vi "App - analyze RUS V6.vi"() -> ()   [LabVIEW 2021] (continued)
"last mod"=timestamp(3493836728 s since 1904-01-01), "file name str"="D:\\Data\\Ultrasound\\LSCO\\LSCO22__130814c\\5_Cooling_2nd_try\\September_2014\\091714\\27.11300K_500_2500_2.10000V_0.00000T_Sep17-2014__18-12-08_001_091714.bin", "mod time(min)"=58230612.13333333, "file format"=enum."binary", "power(V)"=2.1, "Magn Field(T) "=0.0}, {"temperature"=27.012, "temperature str"="27.01200", "file path"=path "D:/Data/Ultrasound/LSCO/LSCO22__130814c/5_Cooling_2nd_try/September_2014/091714/27.01200K_500_2500_2.10000V_0.00000T_Sep17-2014__18-13-27_001_091714.bin", "last mod"=timestamp(3493836807 s since 1904-01-01), "file name str"="D:\\Data\\Ultrasound\\LSCO\\LSCO22__130814c\\5_Cooling_2nd_try\\September_2014\\091714\\27.01200K_500_2500_2.10000V_0.00000T_Sep17-2014__18-13-27_001_091714.bin", "mod time(min)"=58230613.45, "file format"=enum."binary", "power(V)"=2.1, "Magn Field(T) "=0.0}, {"temperature"=26.919, "temperature str"="26.91900", "file path"=path "D:/Data/Ultrasound/LSCO/LSCO22__130814c/5_Cooling_2nd_try/September_2014/091714/26.91900K_500_2500_2.10000V_0.00000T_Sep17-2014__18-14-46_001_091714.bin", "last mod"=timestamp(3493836886 s since 1904-01-01), "file name str"="D:\\Data\\Ultrasound\\LSCO\\LSCO22__130814c\\5_Cooling_2nd_try\\September_2014\\091714\\26.91900K_500_2500_2.10000V_0.00000T_Sep17-2014__18-14-46_001_091714.bin", "mod time(min)"=58230614.766666666, "file format"=enum."binary", "power(V)"=2.1, "Magn Field(T) "=0.0}, {"temperature"=26.829, "temperature str"="26.82900", "file path"=path "D:/Data/Ultrasound/LSCO/LSCO22__130814c/5_Cooling_2nd_try/September_2014/091714/26.82900K_500_2500_2.10000V_0.00000T_Sep17-2014__18-16-06_001_091714.bin", "last mod"=timestamp(3493836966 s since 1904-01-01), "file name str"="D:\\Data\\Ultrasound\\LSCO\\LSCO22__130814c\\5_Cooling_2nd_try\\September_2014\\091714\\26.82900K_500_2500_2.10000V_0.00000T_Sep17-2014__18-16-06_001_091714.bin", "mod time(min)"=58230616.1, "file format"=enum."binary", "power(V)"=2.1, "Magn Field(T) "=0.0}, {"temperature"=26.729, "temperature str"="26.72900", "file path"=path "D:/Data/Ultrasound/LSCO/LSCO22__130814c/5_Cooling_2nd_try/September_2014/091714/26.72900K_500_2500_2.10000V_0.00000T_Sep17-2014__18-17-25_001_091714.bin", "last mod"=timestamp(3493837045 s since 1904-01-01), "file name str"="D:\\Data\\Ultrasound\\LSCO\\LSCO22__130814c\\5_Cooling_2nd_try\\September_2014\\091714\\26.72900K_500_2500_2.10000V_0.00000T_Sep17-2014__18-17-25_001_091714.bin", "mod time(min)"=58230617.416666664, "file format"=enum."binary", "power(V)"=2.1, "Magn Field(T) "=0.0}, {"temperature"=26.631, "temperature str"="26.63100", "file path"=path "D:/Data/Ultrasound/LSCO/LSCO22__130814c/5_Cooling_2nd_try/September_2014/091714/26.63100K_500_2500_2.10000V_0.00000T_Sep17-2014__18-18-44_001_091714.bin", "last mod"=timestamp(3493837124 s since 1904-01-01), "file name str"="D:\\Data\\Ultrasound\\LSCO\\LSCO22__130814c\\5_Cooling_2nd_try\\September_2014\\091714\\26.63100K_500_2500_2.10000V_0.00000T_Sep17-2014__18-18-44_001_091714.bin", "mod time(min)"=58230618.733333334, "file format"=enum."binary", "power(V)"=2.1, "Magn Field(T) "=0.0}, {"temperature"=26.532, "temperature str"="26.53200", "file path"=path "D:/Data/Ultrasound/LSCO/LSCO22__130814c/5_Cooling_2nd_try/September_2014/091714/26.53200K_500_2500_2.10000V_0.00000T_Sep17-2014__18-20-04_001_091714.bin", "last mod"=timestamp(3493837204 s since 1904-01-01), "file name str"="D:\\Data\\Ultrasound\\LSCO\\LSCO22__130814c\\5_Cooling_2nd_try\\September_2014\\091714\\26.53200K_500_2500_2.10000V_0.00000T_Sep17-2014__18-20-04_001_091714.bin", "mod time(min)"=58230620.06666667, "file format"=enum."binary", "power(V)"=2.1, "Magn Field(T) "=0.0}, {"temperature"=26.444, "temperature str"="26.44400", "file path"=path "D:/Data/Ultrasound/LSCO/LSCO22__130814c/5_Cooling_2nd_try/September_2014/091714/26.44400K_500_2500_2.10000V_0.00000T_Sep17-2014__18-21-23_001_091714.bin", "last mod"=timestamp(3493837283 s since 1904-01-01), "file name str"="D:\\Data\\Ultrasound\\LSCO\\LSCO22__130814c\\5_Cooling_2nd_try\\September_2014\\091714\\26.44400K_500_2500_2.10000V_0.00000T_Sep17-2014__18-21-23_001_091714.bin", "mod time(min)"=58230621.38333333, "file format"=enum."binary", "power(V)"=2.1, "Magn Field(T) "=0.0}, {"temperature"=26.344, "temperature str"="26.34400", "file path"=path "D:/Data/Ultrasound/LSCO/LSCO22__130814c/5_Cooling_2nd_try/September_2014/091714/26.34400K_500_2500_2.10000V_0.00000T_Sep17-2014__18-22-43_001_091714.bin", "last mod"=timestamp(3493837363 s since 1904-01-01), "file name str"="D:\\Data\\Ultrasound\\LSCO\\LSCO22__130814c\\5_Cooling_2nd_try\\September_2014\\091714\\26.34400K_500_2500_2.10000V_0.00000T_Sep17-2014__18-22-43_001_091714.bin", "mod time(min)"=58230622.71666667, "file format"=enum."binary", "power(V)"=2.1, "Magn Field(T) "=0.0}, {"temperature"=26.256, "temperature str"="26.25600", "file path"=path "D:/Data/Ultrasound/LSCO/LSCO22__130814c/5_Cooling_2nd_try/September_2014/091714/26.25600K_500_2500_2.10000V_0.00000T_Sep17-2014__18-24-02_001_091714.bin", "last mod"=timestamp(3493837442 s since 1904-01-01), "file name str"="D:\\Data\\Ultrasound\\LSCO\\LSCO22__130814c\\5_Cooling_2nd_try\\September_2014\\091714\\26.25600K_500_2500_2.10000V_0.00000T_Sep17-2014__18-24-02_001_091714.bin", "mod time(min)"=58230624.03333333, "file format"=enum."binary", "power(V)"=2.1, "Magn Field(T) "=0.0}, {"temperature"=26.156, "temperature str"="26.15600", "file path"=path "D:/Data/Ultrasound/LSCO/LSCO22__130814c/5_Cooling_2nd_try/September_2014/091714/26.15600K_500_2500_2.10000V_0.00000T_Sep17-2014__18-25-21_001_091714.bin", "last mod"=timestamp(3493837521 s since 1904-01-01), "file name str"="D:\\Data\\Ultrasound\\LSCO\\LSCO22__130814c\\5_Cooling_2nd_try\\September_2014\\091714\\26.15600K_500_2500_2.10000V_0.00000T_Sep17-2014__18-25-21_001_091714.bin", "mod time(min)"=58230625.35, "file format"=enum."binary", "power(V)"=2.1, "Magn Field(T) "=0.0}, {"temperature"=26.051, "temperature str"="26.05100", "file path"=path "D:/Data/Ultrasound/LSCO/LSCO22__130814c/5_Cooling_2nd_try/September_2014/091714/26.05100K_500_2500_2.10000V_0.00000T_Sep17-2014__18-26-41_001_091714.bin", "last mod"=timestamp(3493837601 s since 1904-01-01), "file name str"="D:\\Data\\Ultrasound\\LSCO\\LSCO22__130814c\\5_Cooling_2nd_try\\September_2014\\091714\\26.05100K_500_2500_2.10000V_0.00000T_Sep17-2014__18-26-41_001_091714.bin", "mod time(min)"=58230626.68333333, "file format"=enum."binary", "power(V)"=2.1, "Magn Field(T) "=0.0}, {"temperature"=25.961, "temperature str"="25.96100", "file path"=path "D:/Data/Ultrasound/LSCO/LSCO22__130814c/5_Cooling_2nd_try/September_2014/091714/25.96100K_500_2500_2.10000V_0.00000T_Sep17-2014__18-28-00_001_091714.bin", "last mod"=timestamp(3493837680 s since 1904-01-01), "file name str"="D:\\Data\\Ultrasound\\LSCO\\LSCO22__130814c\\5_Cooling_2nd_try\\September_2014\\091714\\25.96100K_500_2500_2.10000V_0.00000T_Sep17-2014__18-28-00_001_091714.bin", "mod time(min)"=58230628.0, "file format"=enum."binary", "power(V)"=2.1, "Magn Field(T) "=0.0}, {"temperature"=25.864, "temperature str"="25.86400", "file path"=path "D:/Data/Ultrasound/LSCO/LSCO22__130814c/5_Cooling_2nd_try/September_2014/091714/25.86400K_500_2500_2.10000V_0.00000T_Sep17-2014__18-29-20_001_091714.bin", "last mod"=timestamp(3493837760 s since 1904-01-01), "file name str"="D:\\Data\\Ultrasound\\LSCO\\LSCO22__130814c\\5_Cooling_2nd_try\\September_2014\\091714\\25.86400K_500_2500_2.10000V_0.00000T_Sep17-2014__18-29-20_001_091714.bin", "mod time(min)"=58230629.333333336, "file format"=enum."binary", "power(V)"=2.1, "Magn Field(T) "=0.0}, {"temperature"=25.765, "temperature str"="25.76500", "file path"=path "D:/Data/Ultrasound/LSCO/LSCO22__130814c/5_Cooling_2nd_try/September_2014/091714/25.76500K_500_2500_2.10000V_0.00000T_Sep17-2014__18-30-39_001_091714.bin", "last mod"=timestamp(3493837839 s since 1904-01-01), "file name str"="D:\\Data\\Ultrasound\\LSCO\\LSCO22__130814c\\5_Cooling_2nd_try\\September_2014\\091714\\25.76500K_500_2500_2.10000V_0.00000T_Sep17-2014__18-30-39_001_091714.bin", "mod time(min)"=58230630.65, "file format"=enum."binary", "power(V)"=2.1, "Magn Field(T) "=0.0}, {"temperature"=25.672, "temperature str"="25.67200", "file path"=path "D:/Data/Ultrasound/LSCO/LSCO22__130814c/5_Cooling_2nd_try/September_2014/091714/25.67200K_500_2500_2.10000V_0.00000T_Sep17-2014__18-31-58_001_091714.bin", "last mod"=timestamp(3493837918 s since 1904-01-01), "file name str"="D:\\Data\\Ultrasound\\LSCO\\LSCO22__130814c\\5_Cooling_2nd_try\\September_2014\\091714\\25.67200K_500_2500_2.10000V_0.00000T_Sep17-2014__18-31-58_001_091714.bin", "mod time(min)"=58230631.96666667, "file format"=enum."binary", "power(V)"=2.1, "Magn Field(T) "=0.0}, {"temperature"=25.576, "temperature str"="25.57600", "file path"=path "D:/Data/Ultrasound/LSCO/LSCO22__130814c/5_Cooling_2nd_try/September_2014/091714/25.57600K_500_2500_2.10000V_0.00000T_Sep17-2014__18-33-18_001_091714.bin", "last mod"=timestamp(3493837998 s since 1904-01-01), "file name str"="D:\\Data\\Ultrasound\\LSCO\\LSCO22__130814c\\5_Cooling_2nd_try\\September_2014\\091714\\25.57600K_500_2500_2.10000V_0.00000T_Sep17-2014__18-33-18_001_091714.bin", "mod time(min)"=58230633.3, "file format"=enum."binary", "power(V)"=2.1, "Magn Field(T) "=0.0}, {"temperature"=25.474, "temperature str"="25.47400", "file path"=path "D:/Data/Ultrasound/LSCO/LSCO22__130814c/5_Cooling_2nd_try/September_2014/091714/25.47400K_500_2500_2.10000V_0.00000T_Sep17-2014__18-34-37_001_091714.bin", "last mod"=timestamp(3493838077 s since 1904-01-01), "file name str"="D:\\Data\\Ultrasound\\LSCO\\LSCO22__130814c\\5_Cooling_2nd_try\\September_2014\\091714\\25.47400K_500_2500_2.10000V_0.00000T_Sep17-2014__18-34-37_001_091714.bin", "mod time(min)"=58230634.61666667, "file format"=enum."binary", "power(V)"=2.1, "Magn Field(T) "=0.0}, {"temperature"=25.388, "temperature str"="25.38800", "file path"=path "D:/Data/Ultrasound/LSCO/LSCO22__130814c/5_Cooling_2nd_try/September_2014/091714/25.38800K_500_2500_2.10000V_0.00000T_Sep17-2014__18-35-56_001_091714.bin", "last mod"=timestamp(3493838156 s since 1904-01-01), "file name str"="D:\\Data\\Ultrasound\\LSCO\\LSCO22__130814c\\5_Cooling_2nd_try\\September_2014\\091714\\25.38800K_500_2500_2.10000V_0.00000T_Sep17-2014__18-35-56_001_091714.bin", "mod time(min)"=58230635.93333333, "file format"=enum."binary", "power(V)"=2.1, "Magn Field(T) "=0.0}, {"temperature"=25.289, "temperature str"="25.28900", "file path"=path "D:/Data/Ultrasound/LSCO/LSCO22__130814c/5_Cooling_2nd_try/September_2014/091714/25.28900K_500_2500_2.10000V_0.00000T_Sep17-2014__18-37-16_001_091714.bin", "last mod"=timestamp(3493838236 s since 1904-01-01), "file name str"="D:\\Data\\Ultrasound\\LSCO\\LSCO22__130814c\\5_Cooling_2nd_try\\September_2014\\091714\\25.28900K_500_2500_2.10000V_0.00000T_Sep17-2014__18-37-16_001_091714.bin", "mod time(min)"=58230637.266666666, "file format"=enum."binary", "power(V)"=2.1, "Magn Field(T) "=0.0}, {"temperature"=25.188, "temperature str"="25.18800", "file path"=path "D:/Data/Ultrasound/LSCO/LSCO22__130814c/5_Cooling_2nd_try/September_2014/091714/25.18800K_500_2500_2.10000V_0.00000T_Sep17-2014__18-38-35_001_091714.bin", "last mod"=timestamp(3493838315 s since 1904-01-01), "file name str"="D:\\Data\\Ultrasound\\LSCO\\LSCO22__130814c\\5_Cooling_2nd_try\\September_2014\\091714\\25.18800K_500_2500_2.10000V_0.00000T_Sep17-2014__18-38-35_001_091714.bin", "mod time(min)"=58230638.583333336, "file format"=enum."binary", "power(V)"=2.1, "Magn Field(T) "=0.0}, {"temperature"=25.098, "temperature str"="25.09800", "file path"=path "D:/Data/Ultrasound/LSCO/LSCO22__130814c/5_Cooling_2nd_try/September_2014/091714/25.09800K_500_2500_2.10000V_0.00000T_Sep17-2014__18-39-55_001_091714.bin", "last mod"=timestamp(3493838395 s since 1904-01-01), "file name str"="D:\\Data\\Ultrasound\\LSCO\\LSCO22__130814c\\5_Cooling_2nd_try\\September_2014\\091714\\25.09800K_500_2500_2.10000V_0.00000T_Sep17-2014__18-39-55_001_091714.bin", "mod time(min)"=58230639.916666664, "file format"=enum."binary", "power(V)"=2.1, "Magn Field(T) "=0.0}, {"temperature"=24.995, "temperature str"="24.99500", "file path"=path "D:/Data/Ultrasound/LSCO/LSCO22__130814c/5_Cooling_2nd_try/September_2014/091714/24.99500K_500_2500_2.10000V_0.00000T_Sep17-2014__18-41-14_001_091714.bin", "last mod"=timestamp(3493838474 s since 1904-01-01), "file name str"="D:\\Data\\Ultrasound\\LSCO\\LSCO22__130814c\\5_Cooling_2nd_try\\September_2014\\091714\\24.99500K_500_2500_2.10000V_0.00000T_Sep17-2014__18-41-14_001_091714.bin", "mod time(min)"=58230641.233333334, "file format"=enum."binary", "power(V)"=2.1, "Magn Field(T) "=0.0}, {"temperature"=24.901, "temperature str"="24.90100", "file path"=path "D:/Data/Ultrasound/LSCO/LSCO22__130814c/5_Cooling_2nd_try/September_2014/091714/24.90100K_500_2500_2.10000V_0.00000T_Sep17-2014__18-42-33_001_091714.bin", "last mod"=timestamp(3493838553 s since 1904-01-01), "file name str"="D:\\Data\\Ultrasound\\LSCO\\LSCO22__130814c\\5_Cooling_2nd_try\\September_2014\\091714\\24.90100K_500_2500_2.10000V_0.00000T_Sep17-2014__18-42-33_001_091714.bin", "mod time(min)"=58230642.55, "file format"=enum."binary", "power(V)"=2.1, "Magn Field(T) "=0.0}, {"temperature"=24.798, "temperature str"="24.79800", "file path"=path "D:/Data/Ultrasound/LSCO/LSCO22__130814c/5_Cooling_2nd_try/September_2014/091714/24.79800K_500_2500_2.10000V_0.00000T_Sep17-2014__18-43-53_001_091714.bin", "last mod"=timestamp(3493838633 s since 1904-01-01), "file name str"="D:\\Data\\Ultrasound\\LSCO\\LSCO22__130814c\\5_Cooling_2nd_try\\September_2014\\091714\\24.79800K_500_2500_2.10000V_0.00000T_Sep17-2014__18-43-53_001_091714.bin", "mod time(min)"=58230643.88333333, "file format"=enum."binary", "power(V)"=2.1, "Magn Field(T) "=0.0}, {"temperature"=24.697, "temperature str"="24.69700", "file path"=path "D:/Data/Ultrasound/LSCO/LSCO22__130814c/5_Cooling_2nd_try/September_2014/091714/24.69700K_500_2500_2.10000V_0.00000T_Sep17-2014__18-45-12_001_091714.bin", "last mod"=timestamp(3493838712 s since 1904-01-01), "file name str"="D:\\Data\\Ultrasound\\LSCO\\LSCO22__130814c\\5_Cooling_2nd_try\\September_2014\\091714\\24.69700K_500_2500_2.10000V_0.00000T_Sep17-2014__18-45-12_001_091714.bin", "mod time(min)"=58230645.2, "file format"=enum."binary", "power(V)"=2.1, "Magn Field(T) "=0.0}, {"temperature"=24.601, "temperature str"="24.60100", "file path"=path "D:/Data/Ultrasound/LSCO/LSCO22__130814c/5_Cooling_2nd_try/September_2014/091714/24.60100K_500_2500_2.10000V_0.00000T_Sep17-2014__18-46-31_001_091714.bin", "last mod"=timestamp(3493838791 s since 1904-01-01), "file name str"="D:\\Data\\Ultrasound\\LSCO\\LSCO22__130814c\\5_Cooling_2nd_try\\September_2014\\091714\\24.60100K_500_2500_2.10000V_0.00000T_Sep17-2014__18-46-31_001_091714.bin", "mod time(min)"=58230646.516666666, "file format"=enum."binary", "power(V)"=2.1, "Magn Field(T) "=0.0}, {"temperature"=24.516, "temperature str"="24.51600", "file path"=path "D:/Data/Ultrasound/LSCO/LSCO22__130814c/5_Cooling_2nd_try/September_2014/091714/24.51600K_500_2500_2.10000V_0.00000T_Sep17-2014__18-47-51_001_091714.bin", "last mod"=timestamp(3493838871 s since 1904-01-01), "file name str"="D:\\Data\\Ultrasound\\LSCO\\LSCO22__130814c\\5_Cooling_2nd_try\\September_2014\\091714\\24.51600K_500_2500_2.10000V_0.00000T_Sep17-2014__18-47-51_001_091714.bin", "mod time(min)"=58230647.85, "file format"=enum."binary", "power(V)"=2.1, "Magn Field(T) "=0.0}, {"temperature"=24.408, "temperature str"="24.40800", "file path"=path "D:/Data/Ultrasound/LSCO/LSCO22__130814c/5_Cooling_2nd_try/September_2014/091714/24.40800K_500_2500_2.10000V_0.00000T_Sep17-2014__18-49-10_001_091714.bin", "last mod"=timestamp(3493838950 s since 1904-01-01), "file name str"="D:\\Data\\Ultrasound\\LSCO\\LSCO22__130814c\\5_Cooling_2nd_try\\September_2014\\091714\\24.40800K_500_2500_2.10000V_0.00000T_Sep17-2014__18-49-10_001_091714.bin", "mod time(min)"=58230649.166666664, "file format"=enum."binary", "power(V)"=2.1, "Magn Field(T) "=0.0}, {"temperature"=24.313, "temperature str"="24.31300", "file path"=path "D:/Data/Ultrasound/LSCO/LSCO22__130814c/5_Cooling_2nd_try/September_2014/091714/24.31300K_500_2500_2.10000V_0.00000T_Sep17-2014__18-50-30_001_091714.bin", "last mod"=timestamp(3493839030 s since 1904-01-01), "file name str"="D:\\Data\\Ultrasound\\LSCO\\LSCO22__130814c\\5_Cooling_2nd_try\\September_2014\\091714\\24.31300K_500_2500_2.10000V_0.00000T_Sep17-2014__18-50-30_001_091714.bin", "mod time(min)"=58230650.5, "file format"=enum."binary", "power(V)"=2.1, "Magn Field(T) "=0.0}, {"temperature"=24.219, "temperature str"="24.21900", "file path"=path "D:/Data/Ultrasound/LSCO/LSCO22__130814c/5_Cooling_2nd_try/September_2014/091714/24.21900K_500_2500_2.10000V_0.00000T_Sep17-2014__18-51-49_001_091714.bin", "last mod"=timestamp(3493839109 s since 1904-01-01), "file name str"="D:\\Data\\Ultrasound\\LSCO\\LSCO22__130814c\\5_Cooling_2nd_try\\September_2014\\091714\\24.21900K_500_2500_2.10000V_0.00000T_Sep17-2014__18-51-49_001_091714.bin", "mod time(min)"=58230651.81666667, "file format"=enum."binary", "power(V)"=2.1, "Magn Field(T) "=0.0}, {"temperature"=24.112, "temperature str"="24.11200", "file path"=path "D:/Data/Ultrasound/LSCO/LSCO22__130814c/5_Cooling_2nd_try/September_2014/091714/24.11200K_500_2500_2.10000V_0.00000T_Sep17-2014__18-53-08_001_091714.bin", "last mod"=timestamp(3493839188 s since 1904-01-01), "file name str"="D:\\Data\\Ultrasound\\LSCO\\LSCO22__130814c\\5_Cooling_2nd_try\\September_2014\\091714\\24.11200K_500_2500_2.10000V_0.00000T_Sep17-2014__18-53-08_001_091714.bin", "mod time(min)"=58230653.13333333, "file format"=enum."binary", "power(V)"=2.1, "Magn Field(T) "=0.0}, {"temperature"=24.023, "temperature str"="24.02300", "file path"=path "D:/Data/Ultrasound/LSCO/LSCO22__130814c/5_Cooling_2nd_try/September_2014/091714/24.02300K_500_2500_2.10000V_0.00000T_Sep17-2014__18-54-28_001_091714.bin", "last mod"=timestamp(3493839268 s since 1904-01-01), "file name str"="D:\\Data\\Ultrasound\\LSCO\\LSCO22__130814c\\5_Cooling_2nd_try\\September_2014\\091714\\24.02300K_500_2500_2.10000V_0.00000T_Sep17-2014__18-54-28_001_091714.bin", "mod time(min)"=58230654.46666667, "file format"=enum."binary", "power(V)"=2.1, "Magn Field(T) "=0.0}, {"temperature"=23.922, "temperature str"="23.92200", "file path"=path "D:/Data/Ultrasound/LSCO/LSCO22__130814c/5_Cooling_2nd_try/September_2014/091714/23.92200K_500_2500_2.10000V_0.00000T_Sep17-2014__18-55-47_001_091714.bin", "last mod"=timestamp(3493839347 s since 1904-01-01), "file name str"="D:\\Data\\Ultrasound\\LSCO\\LSCO22__130814c\\5_Cooling_2nd_try\\September_2014\\091714\\23.92200K_500_2500_2.10000V_0.00000T_Sep17-2014__18-55-47_001_091714.bin", "mod time(min)"=58230655.78333333, "file format"=enum."binary", "power(V)"=2.1, "Magn Field(T) "=0.0}, {"temperature"=23.825, "temperature str"="23.82500", "file path"=path "D:/Data/Ultrasound/LSCO/LSCO22__130814c/5_Cooling_2nd_try/September_2014/091714/23.82500K_500_2500_2.10000V_0.00000T_Sep17-2014__18-57-07_001_091714.bin", "last mod"=timestamp(3493839427 s since 1904-01-01), "file name str"="D:\\Data\\Ultrasound\\LSCO\\LSCO22__130814c\\5_Cooling_2nd_try\\September_2014\\091714\\23.82500K_500_2500_2.10000V_0.00000T_Sep17-2014__18-57-07_001_091714.bin", "mod time(min)"=58230657.11666667, "file format"=enum."binary", "power(V)"=2.1, "Magn Field(T) "=0.0}, {"temperature"=23.731, "temperature str"="23.73100", "file path"=path "D:/Data/Ultrasound/LSCO/LSCO22__130814c/5_Cooling_2nd_try/September_2014/091714/23.73100K_500_2500_2.10000V_0.00000T_Sep17-2014__18-58-26_001_091714.bin", "last mod"=timestamp(3493839506 s since 1904-01-01), "file name str"="D:\\Data\\Ultrasound\\LSCO\\LSCO22__130814c\\5_Cooling_2nd_try\\September_2014\\091714\\23.73100K_500_2500_2.10000V_0.00000T_Sep17-2014__18-58-26_001_091714.bin", "mod time(min)"=58230658.43333333, "file format"=enum."binary", "power(V)"=2.1, "Magn Field(T) "=0.0}, {"temperature"=23.634, "temperature str"="23.63400", "file path"=path "D:/Data/Ultrasound/LSCO/LSCO22__130814c/5_Cooling_2nd_try/September_2014/091714/23.63400K_500_2500_2.10000V_0.00000T_Sep17-2014__18-59-45_001_091714.bin", "last mod"=timestamp(3493839585 s since 1904-01-01), "file name str"="D:\\Data\\Ultrasound\\LSCO\\LSCO22__130814c\\5_Cooling_2nd_try\\September_2014\\091714\\23.63400K_500_2500_2.10000V_0.00000T_Sep17-2014__18-59-45_001_091714.bin", "mod time(min)"=58230659.75, "file format"=enum."binary", "power(V)"=2.1, "Magn Field(T) "=0.0}, {"temperature"=23.53, "temperature str"="23.53000", "file path"=path "D:/Data/Ultrasound/LSCO/LSCO22__130814c/5_Cooling_2nd_try/September_2014/091714/23.53000K_500_2500_2.10000V_0.00000T_Sep17-2014__19-01-05_001_091714.bin", "last mod"=timestamp(3493839665 s since 1904-01-01), "file name str"="D:\\Data\\Ultrasound\\LSCO\\LSCO22__130814c\\5_Cooling_2nd_try\\September_2014\\091714\\23.53000K_500_2500_2.10000V_0.00000T_Sep17-2014__19-01-05_001_091714.bin", "mod time(min)"=58230661.083333336, "file format"=enum."binary", "power(V)"=2.1, "Magn Field(T) "=0.0}, {"temperature"=23.436, "temperature str"="23.43600", "file path"=path "D:/Data/Ultrasound/LSCO/LSCO22__130814c/5_Cooling_2nd_try/September_2014/091714/23.43600K_500_2500_2.10000V_0.00000T_Sep17-2014__19-02-24_001_091714.bin", "last mod"=timestamp(3493839744 s since 1904-01-01), "file name str"="D:\\Data\\Ultrasound\\LSCO\\LSCO22__130814c\\5_Cooling_2nd_try\\September_2014\\091714\\23.43600K_500_2500_2.10000V_0.00000T_Sep17-2014__19-02-24_001_091714.bin", "mod time(min)"=58230662.4, "file format"=enum."binary", "power(V)"=2.1, "Magn Field(T) "=0.0}, {"temperature"=23.334, "temperature str"="23.33400", "file path"=path "D:/Data/Ultrasound/LSCO/LSCO22__130814c/5_Cooling_2nd_try/September_2014/091714/23.33400K_500_2500_2.10000V_0.00000T_Sep17-2014__19-03-43_001_091714.bin", "last mod"=timestamp(3493839823 s since 1904-01-01), "file name str"="D:\\Data\\Ultrasound\\LSCO\\LSCO22__130814c\\5_Cooling_2nd_try\\September_2014\\091714\\23.33400K_500_2500_2.10000V_0.00000T_Sep17-2014__19-03-43_001_091714.bin", "mod time(min)"=58230663.71666667, "file format"=enum."binary", "power(V)"=2.1, "Magn Field(T) "=0.0}, {"temperature"=23.235, "temperature str"="23.23500", "file path"=path "D:/Data/Ultrasound/LSCO/LSCO22__130814c/5_Cooling_2nd_try/September_2014/091714/23.23500K_500_2500_2.10000V_0.00000T_Sep17-2014__19-05-03_001_091714.bin", "last mod"=timestamp(3493839903 s since 1904-01-01), "file name str"="D:\\Data\\Ultrasound\\LSCO\\LSCO22__130814c\\5_Cooling_2nd_try\\September_2014\\091714\\23.23500K_500_2500_2.10000V_0.00000T_Sep17-2014__19-05-03_001_091714.bin", "mod time(min)"=58230665.05, "file format"=enum."binary", "power(V)"=2.1, "Magn Field(T) "=0.0}, {"temperature"=23.139, "temperature str"="23.13900", "file path"=path "D:/Data/Ultrasound/LSCO/LSCO22__130814c/5_Cooling_2nd_try/September_2014/091714/23.13900K_500_2500_2.10000V_0.00000T_Sep17-2014__19-06-22_001_091714.bin", "last mod"=timestamp(3493839982 s since 1904-01-01), "file name str"="D:\\Data\\Ultrasound\\LSCO\\LSCO22__130814c\\5_Cooling_2nd_try\\September_2014\\091714\\23.13900K_500_2500_2.10000V_0.00000T_Sep17-2014__19-06-22_001_091714.bin", "mod time(min)"=58230666.36666667, "file format"=enum."binary", "power(V)"=2.1, "Magn Field(T) "=0.0}, {"temperature"=23.041, "temperature str"="23.04100", "file path"=path "D:/Data/Ultrasound/LSCO/LSCO22__130814c/5_Cooling_2nd_try/September_2014/091714/23.04100K_500_2500_2.10000V_0.00000T_Sep17-2014__19-07-42_001_091714.bin", "last mod"=timestamp(3493840062 s since 1904-01-01), "file name str"="D:\\Data\\Ultrasound\\LSCO\\LSCO22__130814c\\5_Cooling_2nd_try\\September_2014\\091714\\23.04100K_500_2500_2.10000V_0.00000T_Sep17-2014__19-07-42_001_091714.bin", "mod time(min)"=58230667.7, "file format"=enum."binary", "power(V)"=2.1, "Magn Field(T) "=0.0}, {"temperature"=22.937, "temperature str"="22.93700", "file path"=path "D:/Data/Ultrasound/LSCO/LSCO22__130814c/5_Cooling_2nd_try/September_2014/091714/22.93700K_500_2500_2.10000V_0.00000T_Sep17-2014__19-09-01_001_091714.bin", "last mod"=timestamp(3493840141 s since 1904-01-01), "file name str"="D:\\Data\\Ultrasound\\LSCO\\LSCO22__130814c\\5_Cooling_2nd_try\\September_2014\\091714\\22.93700K_500_2500_2.10000V_0.00000T_Sep17-2014__19-09-01_001_091714.bin", "mod time(min)"=58230669.016666666, "file format"=enum."binary", "power(V)"=2.1, "Magn Field(T) "=0.0}, {"temperature"=22.842, "temperature str"="22.84200", "file path"=path "D:/Data/Ultrasound/LSCO/LSCO22__130814c/5_Cooling_2nd_try/September_2014/091714/22.84200K_500_2500_2.10000V_0.00000T_Sep17-2014__19-10-20_001_091714.bin", "last mod"=timestamp(3493840220 s since 1904-01-01), "file name str"="D:\\Data\\Ultrasound\\LSCO\\LSCO22__130814c\\5_Cooling_2nd_try\\September_2014\\091714\\22.84200K_500_2500_2.10000V_0.00000T_Sep17-2014__19-10-20_001_091714.bin", "mod time(min)"=58230670.333333336, "file format"=enum."binary", "power(V)"=2.1, "Magn Field(T) "=0.0}, {"temperature"=22.748, "temperature str"="22.74800", "file path"=path "D:/Data/Ultrasound/LSCO/LSCO22__130814c/5_Cooling_2nd_try/September_2014/091714/22.74800K_500_2500_2.10000V_0.00000T_Sep17-2014__19-11-40_001_091714.bin", "last mod"=timestamp(3493840300 s since 1904-01-01), "file name str"="D:\\Data\\Ultrasound\\LSCO\\LSCO22__130814c\\5_Cooling_2nd_try\\September_2014\\091714\\22.74800K_500_2500_2.10000V_0.00000T_Sep17-2014__19-11-40_001_091714.bin", "mod time(min)"=58230671.666666664, "file format"=enum."binary", "power(V)"=2.1, "Magn Field(T) "=0.0}, {"temperature"=22.644, "temperature str"="22.64400", "file path"=path "D:/Data/Ultrasound/LSCO/LSCO22__130814c/5_Cooling_2nd_try/September_2014/091714/22.64400K_500_2500_2.10000V_0.00000T_Sep17-2014__19-12-59_001_091714.bin", "last mod"=timestamp(3493840379 s since 1904-01-01), "file name str"="D:\\Data\\Ultrasound\\LSCO\\LSCO22__130814c\\5_Cooling_2nd_try\\September_2014\\091714\\22.64400K_500_2500_2.10000V_0.00000T_Sep17-2014__19-12-59_001_091714.bin", "mod time(min)"=58230672.983333334, "file format"=enum."binary", "power(V)"=2.1, "Magn Field(T) "=0.0}, {"temperature"=22.549, "temperature str"="22.54900", "file path"=path "D:/Data/Ultrasound/LSCO/LSCO22__130814c/5_Cooling_2nd_try/September_2014/091714/22.54900K_500_2500_2.10000V_0.00000T_Sep17-2014__19-14-18_001_091714.bin", "last mod"=timestamp(3493840458 s since 1904-01-01), "file name str"="D:\\Data\\Ultrasound\\LSCO\\LSCO22__130814c\\5_Cooling_2nd_try\\September_2014\\091714\\22.54900K_500_2500_2.10000V_0.00000T_Sep17-2014__19-14-18_001_091714.bin", "mod time(min)"=58230674.3, "file format"=enum."binary", "power(V)"=2.1, "Magn Field(T) "=0.0}, {"temperature"=22.448, "temperature str"="22.44800", "file path"=path "D:/Data/Ultrasound/LSCO/LSCO22__130814c/5_Cooling_2nd_try/September_2014/091714/22.44800K_500_2500_2.10000V_0.00000T_Sep17-2014__19-15-38_001_091714.bin", "last mod"=timestamp(3493840538 s since 1904-01-01), "file name str"="D:\\Data\\Ultrasound\\LSCO\\LSCO22__130814c\\5_Cooling_2nd_try\\September_2014\\091714\\22.44800K_500_2500_2.10000V_0.00000T_Sep17-2014__19-15-38_001_091714.bin", "mod time(min)"=58230675.63333333, "file format"=enum."binary", "power(V)"=2.1, "Magn Field(T) "=0.0}, {"temperature"=22.345, "temperature str"="22.34500", "file path"=path "D:/Data/Ultrasound/LSCO/LSCO22__130814c/5_Cooling_2nd_try/September_2014/091714/22.34500K_500_2500_2.10000V_0.00000T_Sep17-2014__19-16-57_001_091714.bin", "last mod"=timestamp(3493840617 s since 1904-01-01), "file name str"="D:\\Data\\Ultrasound\\LSCO\\LSCO22__130814c\\5_Cooling_2nd_try\\September_2014\\091714\\22.34500K_500_2500_2.10000V_0.00000T_Sep17-2014__19-16-57_001_091714.bin", "mod time(min)"=58230676.95, "file format"=enum."binary", "power(V)"=2.1, "Magn Field(T) "=0.0}, {"temperature"=22.254, "temperature str"="22.25400", "file path"=path "D:/Data/Ultrasound/LSCO/LSCO22__130814c/5_Cooling_2nd_try/September_2014/091714/22.25400K_500_2500_2.10000V_0.00000T_Sep17-2014__19-18-17_001_091714.bin", "last mod"=timestamp(3493840697 s since 1904-01-01), "file name str"="D:\\Data\\Ultrasound\\LSCO\\LSCO22__130814c\\5_Cooling_2nd_try\\September_2014\\091714\\22.25400K_500_2500_2.10000V_0.00000T_Sep17-2014__19-18-17_001_091714.bin", "mod time(min)"=58230678.28333333, "file format"=enum."binary", "power(V)"=2.1, "Magn Field(T) "=0.0}, {"temperature"=22.148, "temperature str"="22.14800", "file path"=path "D:/Data/Ultrasound/LSCO/LSCO22__130814c/5_Cooling_2nd_try/September_2014/091714/22.14800K_500_2500_2.10000V_0.00000T_Sep17-2014__19-19-36_001_091714.bin", "last mod"=timestamp(3493840776 s since 1904-01-01), "file name str"="D:\\Data\\Ultrasound\\LSCO\\LSCO22__130814c\\5_Cooling_2nd_try\\September_2014\\091714\\22.14800K_500_2500_2.10000V_0.00000T_Sep17-2014__19-19-36_001_091714.bin", "mod time(min)"=58230679.6, "file format"=enum."binary", "power(V)"=2.1, "Magn Field(T) "=0.0}, {"temperature"=22.046, "temperature str"="22.04600", "file path"=path "D:/Data/Ultrasound/LSCO/LSCO22__130814c/5_Cooling_2nd_try/September_2014/091714/22.04600K_500_2500_2.10000V_0.00000T_Sep17-2014__19-20-55_001_091714.bin", "last mod"=timestamp(3493840855 s since 1904-01-01), "file name str"="D:\\Data\\Ultrasound\\LSCO\\LSCO22__130814c\\5_Cooling_2nd_try\\September_2014\\091714\\22.04600K_500_2500_2.10000V_0.00000T_Sep17-2014__19-20-55_001_091714.bin", "mod time(min)"=58230680.916666664, "file format"=enum."binary", "power(V)"=2.1, "Magn Field(T) "=0.0}, {"temperature"=21.957, "temperature str"="21.95700", "file path"=path "D:/Data/Ultrasound/LSCO/LSCO22__130814c/5_Cooling_2nd_try/September_2014/091714/21.95700K_500_2500_2.10000V_0.00000T_Sep17-2014__19-22-15_001_091714.bin", "last mod"=timestamp(3493840935 s since 1904-01-01), "file name str"="D:\\Data\\Ultrasound\\LSCO\\LSCO22__130814c\\5_Cooling_2nd_try\\September_2014\\091714\\21.95700K_500_2500_2.10000V_0.00000T_Sep17-2014__19-22-15_001_091714.bin", "mod time(min)"=58230682.25, "file format"=enum."binary", "power(V)"=2.1, "Magn Field(T) "=0.0}, {"temperature"=21.851, "temperature str"="21.85100", "file path"=path "D:/Data/Ultrasound/LSCO/LSCO22__130814c/5_Cooling_2nd_try/September_2014/091714/21.85100K_500_2500_2.10000V_0.00000T_Sep17-2014__19-23-34_001_091714.bin", "last mod"=timestamp(3493841014 s since 1904-01-01), "file name str"="D:\\Data\\Ultrasound\\LSCO\\LSCO22__130814c\\5_Cooling_2nd_try\\September_2014\\091714\\21.85100K_500_2500_2.10000V_0.00000T_Sep17-2014__19-23-34_001_091714.bin", "mod time(min)"=58230683.56666667, "file format"=enum."binary", "power(V)"=2.1, "Magn Field(T) "=0.0}, {"temperature"=21.755, "temperature str"="21.75500", "file path"=path "D:/Data/Ultrasound/LSCO/LSCO22__130814c/5_Cooling_2nd_try/September_2014/091714/21.75500K_500_2500_2.10000V_0.00000T_Sep17-2014__19-24-54_001_091714.bin", "last mod"=timestamp(3493841094 s since 1904-01-01), "file name str"="D:\\Data\\Ultrasound\\LSCO\\LSCO22__130814c\\5_Cooling_2nd_try\\September_2014\\091714\\21.75500K_500_2500_2.10000V_0.00000T_Sep17-2014__19-24-54_001_091714.bin", "mod time(min)"=58230684.9, "file format"=enum."binary", "power(V)"=2.1, "Magn Field(T) "=0.0}, {"temperature"=21.657, "temperature str"="21.65700", "file path"=path "D:/Data/Ultrasound/LSCO/LSCO22__130814c/5_Cooling_2nd_try/September_2014/091714/21.65700K_500_2500_2.10000V_0.00000T_Sep17-2014__19-26-13_001_091714.bin", "last mod"=timestamp(3493841173 s since 1904-01-01), "file name str"="D:\\Data\\Ultrasound\\LSCO\\LSCO22__130814c\\5_Cooling_2nd_try\\September_2014\\091714\\21.65700K_500_2500_2.10000V_0.00000T_Sep17-2014__19-26-13_001_091714.bin", "mod time(min)"=58230686.21666667, "file format"=enum."binary", "power(V)"=2.1, "Magn Field(T) "=0.0}, {"temperature"=21.553, "temperature str"="21.55300", "file path"=path "D:/Data/Ultrasound/LSCO/LSCO22__130814c/5_Cooling_2nd_try/September_2014/091714/21.55300K_500_2500_2.10000V_0.00000T_Sep17-2014__19-27-32_001_091714.bin", "last mod"=timestamp(3493841252 s since 1904-01-01), "file name str"="D:\\Data\\Ultrasound\\LSCO\\LSCO22__130814c\\5_Cooling_2nd_try\\September_2014\\091714\\21.55300K_500_2500_2.10000V_0.00000T_Sep17-2014__19-27-32_001_091714.bin", "mod time(min)"=58230687.53333333, "file format"=enum."binary", "power(V)"=2.1, "Magn Field(T) "=0.0}, {"temperature"=21.455, "temperature str"="21.45500", "file path"=path "D:/Data/Ultrasound/LSCO/LSCO22__130814c/5_Cooling_2nd_try/September_2014/091714/21.45500K_500_2500_2.10000V_0.00000T_Sep17-2014__19-28-52_001_091714.bin", "last mod"=timestamp(3493841332 s since 1904-01-01), "file name str"="D:\\Data\\Ultrasound\\LSCO\\LSCO22__130814c\\5_Cooling_2nd_try\\September_2014\\091714\\21.45500K_500_2500_2.10000V_0.00000T_Sep17-2014__19-28-52_001_091714.bin", "mod time(min)"=58230688.86666667, "file format"=enum."binary", "power(V)"=2.1, "Magn Field(T) "=0.0}, {"temperature"=21.36, "temperature str"="21.36000", "file path"=path "D:/Data/Ultrasound/LSCO/LSCO22__130814c/5_Cooling_2nd_try/September_2014/091714/21.36000K_500_2500_2.10000V_0.00000T_Sep17-2014__19-30-11_001_091714.bin", "last mod"=timestamp(3493841411 s since 1904-01-01), "file name str"="D:\\Data\\Ultrasound\\LSCO\\LSCO22__130814c\\5_Cooling_2nd_try\\September_2014\\091714\\21.36000K_500_2500_2.10000V_0.00000T_Sep17-2014__19-30-11_001_091714.bin", "mod time(min)"=58230690.18333333, "file format"=enum."binary", "power(V)"=2.1, "Magn Field(T) "=0.0}, {"temperature"=21.259, "temperature str"="21.25900", "file path"=path "D:/Data/Ultrasound/LSCO/LSCO22__130814c/5_Cooling_2nd_try/September_2014/091714/21.25900K_500_2500_2.10000V_0.00000T_Sep17-2014__19-31-30_001_091714.bin", "last mod"=timestamp(3493841490 s since 1904-01-01), "file name str"="D:\\Data\\Ultrasound\\LSCO\\LSCO22__130814c\\5_Cooling_2nd_try\\September_2014\\091714\\21.25900K_500_2500_2.10000V_0.00000T_Sep17-2014__19-31-30_001_091714.bin", "mod time(min)"=58230691.5, "file format"=enum."binary", "power(V)"=2.1, "Magn Field(T) "=0.0}, {"temperature"=21.158, "temperature str"="21.15800", "file path"=path "D:/Data/Ultrasound/LSCO/LSCO22__130814c/5_Cooling_2nd_try/September_2014/091714/21.15800K_500_2500_2.10000V_0.00000T_Sep17-2014__19-32-50_001_091714.bin", "last mod"=timestamp(3493841570 s since 1904-01-01), "file name str"="D:\\Data\\Ultrasound\\LSCO\\LSCO22__130814c\\5_Cooling_2nd_try\\September_2014\\091714\\21.15800K_500_2500_2.10000V_0.00000T_Sep17-2014__19-32-50_001_091714.bin", "mod time(min)"=58230692.833333336, "file format"=enum."binary", "power(V)"=2.1, "Magn Field(T) "=0.0}, {"temperature"=21.06, "temperature str"="21.06000", "file path"=path "D:/Data/Ultrasound/LSCO/LSCO22__130814c/5_Cooling_2nd_try/September_2014/091714/21.06000K_500_2500_2.10000V_0.00000T_Sep17-2014__19-34-09_001_091714.bin", "last mod"=timestamp(3493841649 s since 1904-01-01), "file name str"="D:\\Data\\Ultrasound\\LSCO\\LSCO22__130814c\\5_Cooling_2nd_try\\September_2014\\091714\\21.06000K_500_2500_2.10000V_0.00000T_Sep17-2014__19-34-09_001_091714.bin", "mod time(min)"=58230694.15, "file format"=enum."binary", "power(V)"=2.1, "Magn Field(T) "=0.0}, {"temperature"=20.959, "temperature str"="20.95900", "file path"=path "D:/Data/Ultrasound/LSCO/LSCO22__130814c/5_Cooling_2nd_try/September_2014/091714/20.95900K_500_2500_2.10000V_0.00000T_Sep17-2014__19-35-29_001_091714.bin", "last mod"=timestamp(3493841729 s since 1904-01-01), "file name str"="D:\\Data\\Ultrasound\\LSCO\\LSCO22__130814c\\5_Cooling_2nd_try\\September_2014\\091714\\20.95900K_500_2500_2.10000V_0.00000T_Sep17-2014__19-35-29_001_091714.bin", "mod time(min)"=58230695.483333334, "file format"=enum."binary", "power(V)"=2.1, "Magn Field(T) "=0.0}, {"temperature"=20.861, "temperature str"="20.86100", "file path"=path "D:/Data/Ultrasound/LSCO/LSCO22__130814c/5_Cooling_2nd_try/September_2014/091714/20.86100K_500_2500_2.10000V_0.00000T_Sep17-2014__19-36-48_001_091714.bin", "last mod"=timestamp(3493841808 s since 1904-01-01), "file name str"="D:\\Data\\Ultrasound\\LSCO\\LSCO22__130814c\\5_Cooling_2nd_try\\September_2014\\091714\\20.86100K_500_2500_2.10000V_0.00000T_Sep17-2014__19-36-48_001_091714.bin", "mod time(min)"=58230696.8, "file format"=enum."binary", "power(V)"=2.1, "Magn Field(T) "=0.0}, {"temperature"=20.758, "temperature str"="20.75800", "file path"=path "D:/Data/Ultrasound/LSCO/LSCO22__130814c/5_Cooling_2nd_try/September_2014/091714/20.75800K_500_2500_2.10000V_0.00000T_Sep17-2014__19-38-07_001_091714.bin", "last mod"=timestamp(3493841887 s since 1904-01-01), "file name str"="D:\\Data\\Ultrasound\\LSCO\\LSCO22__130814c\\5_Cooling_2nd_try\\September_2014\\091714\\20.75800K_500_2500_2.10000V_0.00000T_Sep17-2014__19-38-07_001_091714.bin", "mod time(min)"=58230698.11666667, "file format"=enum."binary", "power(V)"=2.1, "Magn Field(T) "=0.0}, {"temperature"=20.654, "temperature str"="20.65400", "file path"=path "D:/Data/Ultrasound/LSCO/LSCO22__130814c/5_Cooling_2nd_try/September_2014/091714/20.65400K_500_2500_2.10000V_0.00000T_Sep17-2014__19-39-27_001_091714.bin", "last mod"=timestamp(3493841967 s since 1904-01-01), "file name str"="D:\\Data\\Ultrasound\\LSCO\\LSCO22__130814c\\5_Cooling_2nd_try\\September_2014\\091714\\20.65400K_500_2500_2.10000V_0.00000T_Sep17-2014__19-39-27_001_091714.bin", "mod time(min)"=58230699.45, "file format"=enum."binary", "power(V)"=2.1, "Magn Field(T) "=0.0}, {"temperature"=20.555, "temperature str"="20.55500", "file path"=path "D:/Data/Ultrasound/LSCO/LSCO22__130814c/5_Cooling_2nd_try/September_2014/091714/20.55500K_500_2500_2.10000V_0.00000T_Sep17-2014__19-40-46_001_091714.bin", "last mod"=timestamp(3493842046 s since 1904-01-01), "file name str"="D:\\Data\\Ultrasound\\LSCO\\LSCO22__130814c\\5_Cooling_2nd_try\\September_2014\\091714\\20.55500K_500_2500_2.10000V_0.00000T_Sep17-2014__19-40-46_001_091714.bin", "mod time(min)"=58230700.766666666, "file format"=enum."binary", "power(V)"=2.1, "Magn Field(T) "=0.0}, {"temperature"=20.461, "temperature str"="20.46100", "file path"=path "D:/Data/Ultrasound/LSCO/LSCO22__130814c/5_Cooling_2nd_try/September_2014/091714/20.46100K_500_2500_2.10000V_0.00000T_Sep17-2014__19-42-05_001_091714.bin", "last mod"=timestamp(3493842125 s since 1904-01-01), "file name str"="D:\\Data\\Ultrasound\\LSCO\\LSCO22__130814c\\5_Cooling_2nd_try\\September_2014\\091714\\20.46100K_500_2500_2.10000V_0.00000T_Sep17-2014__19-42-05_001_091714.bin", "mod time(min)"=58230702.083333336, "file format"=enum."binary", "power(V)"=2.1, "Magn Field(T) "=0.0}, {"temperature"=20.355, "temperature str"="20.35500", "file path"=path "D:/Data/Ultrasound/LSCO/LSCO22__130814c/5_Cooling_2nd_try/September_2014/091714/20.35500K_500_2500_2.10000V_0.00000T_Sep17-2014__19-43-25_001_091714.bin", "last mod"=timestamp(3493842205 s since 1904-01-01), "file name str"="D:\\Data\\Ultrasound\\LSCO\\LSCO22__130814c\\5_Cooling_2nd_try\\September_2014\\091714\\20.35500K_500_2500_2.10000V_0.00000T_Sep17-2014__19-43-25_001_091714.bin", "mod time(min)"=58230703.416666664, "file format"=enum."binary", "power(V)"=2.1, "Magn Field(T) "=0.0}, {"temperature"=20.262, "temperature str"="20.26200", "file path"=path "D:/Data/Ultrasound/LSCO/LSCO22__130814c/5_Cooling_2nd_try/September_2014/091714/20.26200K_500_2500_2.10000V_0.00000T_Sep17-2014__19-44-44_001_091714.bin", "last mod"=timestamp(3493842284 s since 1904-01-01), "file name str"="D:\\Data\\Ultrasound\\LSCO\\LSCO22__130814c\\5_Cooling_2nd_try\\September_2014\\091714\\20.26200K_500_2500_2.10000V_0.00000T_Sep17-2014__19-44-44_001_091714.bin", "mod time(min)"=58230704.733333334, "file format"=enum."binary", "power(V)"=2.1, "Magn Field(T) "=0.0}, {"temperature"=20.157, "temperature str"="20.15700", "file path"=path "D:/Data/Ultrasound/LSCO/LSCO22__130814c/5_Cooling_2nd_try/September_2014/091714/20.15700K_500_2500_2.10000V_0.00000T_Sep17-2014__19-46-04_001_091714.bin", "last mod"=timestamp(3493842364 s since 1904-01-01), "file name str"="D:\\Data\\Ultrasound\\LSCO\\LSCO22__130814c\\5_Cooling_2nd_try\\September_2014\\091714\\20.15700K_500_2500_2.10000V_0.00000T_Sep17-2014__19-46-04_001_091714.bin", "mod time(min)"=58230706.06666667, 
